vi "DHE_DRV_close_driver.vi"(0 "fd":i32, 11 "error in (no error)":errorcluster) -> (15 "error out":errorcluster)   [LabVIEW 2016]
doc: "This VI closes the I/O interface with the instrument."
uses:
  c/lib/libarcDHE.so
panel:
  out "error_code":i32
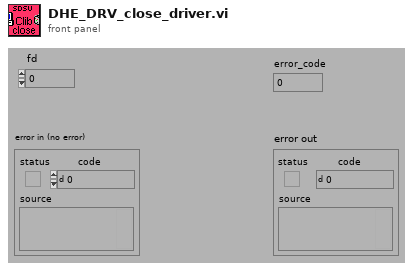
[diagram p1: front panel]
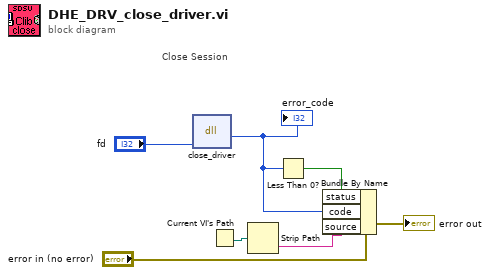
[diagram p0: block diagram]
diagram:
  # "Close Session"
  n1 = dll-call lib="home/simager/panview/PAN/Modules/SDSU/private/c/lib/libarcDHE.so" fn="close_driver"("fd"="fd") -> (w4:i32)  [unwired: 4 in, 2 out]
  "error_code" <- w4
  n2 = Current VI's Path() -> (path=w3:path)
  n3 = Strip Path(path=w3) -> (name=w2:string)  [unwired: 1 out]
  n4 = Less Than 0?(x=w4) -> (x < 0?=w5:bool)
  n5 = Bundle By Name(cluster="error in (no error)", "status"=w5, "code"=w4, "source"=w2) -> (→"error out":errorcluster)
